vi "filelist_datetime.vi"(8 "error in":errorcluster, 11 "cl_filename_pathout":cluster{"filename":string, "arr_pathout":path}[](array[cluster])) -> (0 "error out":errorcluster, 3 "arr_cl_lastmod_path":T1(array[cluster]))   [LabVIEW 2026]
uses:
  <vilib>/Utility/miscctls.llb/LVDateTimeRec.ctl
panel:
  out "arr_cl_lastmod":T2[](array[typedef])
  out "last mod":timestamp[](array[timestamp])
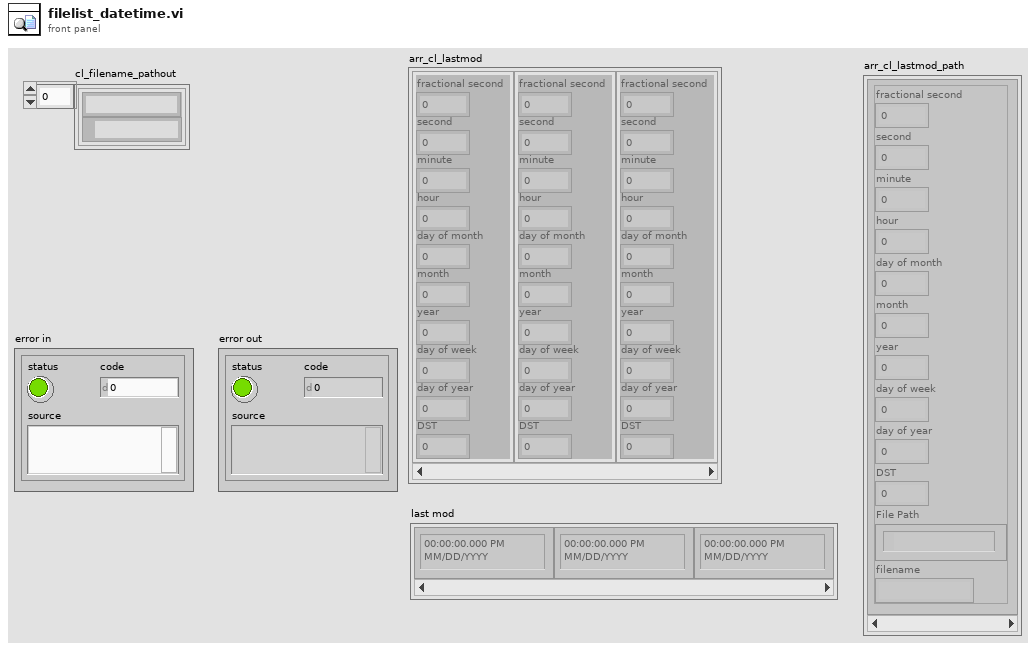
[diagram p1: front panel]
types:
  T1 = cluster{"File Path":path, "DST":i32, "day of year":i32, "day of week":i32, "year":i32, "month":i32, "day of month":i32, "hour":i32, "minute":i32, "second":i32, "fractional second":dbl, "filename":string}[]
  T2 = typedef "LVDateTimeRec.ctl" = cluster{"fractional second":dbl, "second":i32, "minute":i32, "hour":i32, "day of month":i32, "month":i32, "year":i32, "day of week":i32, "day of year":i32, "DST":i32}
  T3 = cluster{"File Path":path, "DST":i32, "day of year":i32, "day of week":i32, "year":i32, "month":i32, "day of month":i32, "hour":i32, "minute":i32, "second":i32, "fractional second":dbl, "filename":string}
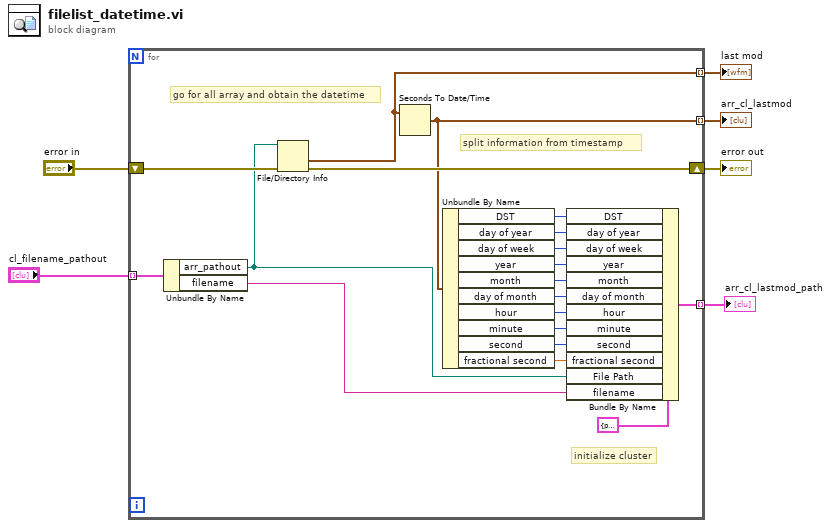
[diagram p0: block diagram]
diagram:
  n1 = for {
    shift-right: [w24] -> w5
    shift-left: "error in" -> [w25]
    tunnel: [w23] -> w4 mode=indexing
    tunnel: [w21] -> w3 mode=indexing
    tunnel: [w22] -> w1 mode=indexing
    tunnel: "cl_filename_pathout" -> [w9] mode=indexing
    # "split information from timestamp"
    # "initialize cluster"
    # "go for all array and obtain the datetime"
    n2 = Unbundle By Name(w9) -> ("arr_pathout"=w8:path, "filename"=w7:string)
    n3 = File/Directory Info(path=w8, error in=w25) -> (last mod=w23:timestamp, error out=w24:errorcluster)  [unwired: 5 out]
    n4 = Seconds To Date/Time(time stamp (now)=w23) -> (date time rec=w21:T2)  [unwired: 1 in]
    n5 = Unbundle By Name(w21) -> ("DST"=w19:i32, "day of year"=w18:i32, "day of week"=w17:i32, "year"=w16:i32, "month"=w15:i32, "day of month"=w14:i32, "hour"=w13:i32, "minute"=w12:i32, "second"=w11:i32, "fractional second"=w20:dbl)
    n6 = Bundle By Name(cluster=T3 {"File Path"=path "", "DST"=0, "day of year"=0, "day of week"=0, "year"=0, "month"=0, "day of month"=0, "hour"=0, "minute"=0, "second"=0, "fractional second"=0.0, "filename"=""} ("arr_cl_lastmod_path"), "DST"=w19, "day of year"=w18, "day of week"=w17, "year"=w16, "month"=w15, "day of month"=w14, "hour"=w13, "minute"=w12, "second"=w11, "fractional second"=w20, "File Path"=w8, "filename"=w7) -> (w22:T3)
  }
  "error out" <- w5
  "last mod" <- w4
  "arr_cl_lastmod" <- w3
  "arr_cl_lastmod_path" <- w1
